vi "MTS_AutoPointCords.vi"(7 "Is Auto Point":bool, 8 "Cords In":T1, 10 "Next Auto Measure Point":i32, 11 "Pattern":dbl[][](array[numeric])) -> (0 "Cords":T1)   [LabVIEW 2010]
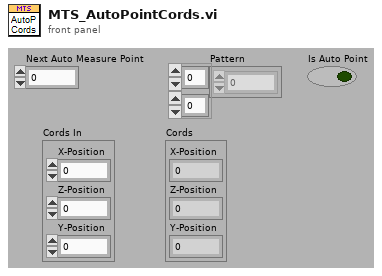
[diagram p1: front panel]
types:
  T1 = cluster{"X-Position":dbl, "Y-Position":dbl, "Z-Position":dbl}
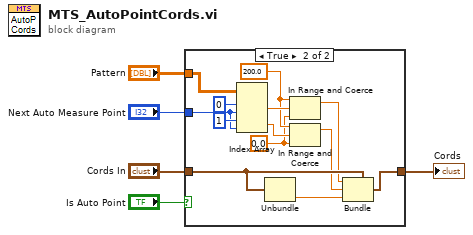
[diagram p0: block diagram]
diagram:
  n1 = case shown="True" "Is Auto Point" {
    tunnel: [w6 w19] -> w5
    tunnel: "Next Auto Measure Point" -> [_ w14]
    tunnel: "Pattern" -> [_ w17]
    tunnel: "Cords In" -> [w6 w18]
    frame False {
    }
    frame True {
      w9 = 0.0 ("lower limit")
      w10 = 200.0 ("upper limit")
      n2 = Index Array(array=w17, index (row) #1=0 ("index (row)"), index (col) #1=w14, index (row) #2=1 ("index (row)"), index (col) #2=w14) -> (element #1=w12:dbl, element #2=w11:dbl)
      n3 = Unbundle(w18) -> ("Z-Position"=w13:dbl)  [unwired: 2 out]
      n4 = In Range and Coerce(upper limit=w10, x=w12, lower limit=w9) -> (coerced(x)=w8:dbl)  [unwired: 1 out]
      n5 = In Range and Coerce(upper limit=w10, x=w11, lower limit=w9) -> (coerced(x)=w7:dbl)  [unwired: 1 out]
      n6 = Bundle(cluster=w18, "X-Position"=w8, "Y-Position"=w7, "Z-Position"=w13) -> (w19:T1)
    }
  }
  "Cords" <- w5
